vi "ReflectiveFunc.vi"(0 "Y":dbl[](array[numeric]), 1 "X":dbl[](array[numeric]), 2 "Coefficients":dbl[](array[numeric])) -> (3 "Y converted":dbl[](array[numeric]), 4 "X converted":dbl[](array[numeric]), 5 "Residue":dbl[](array[numeric]), 6 "f(X,a)":dbl[](array[numeric]))   [LabVIEW 2020, in "XYcenter.lvlib"]
uses:
  XYcenter.lvlib
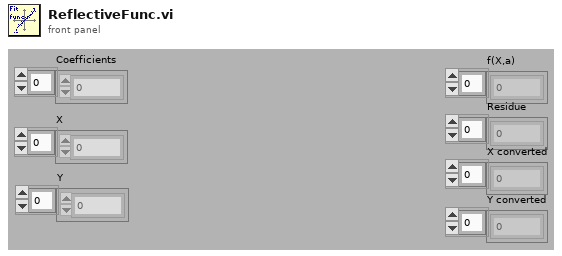
[diagram p1: front panel]
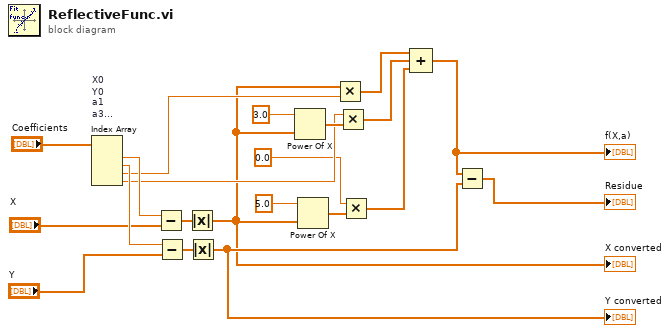
[diagram p0: block diagram]
diagram:
  n1 = Index Array "X0\nY0\na1\na3\na5"(array="Coefficients") -> (element #1=w17:dbl, element #2=w18:dbl, element #3=w7:dbl, element #4=w6:dbl)  [unwired: 4 in]
  n2 = Subtract(x=w17, y="X") -> (x-y=w20:dbl[])
  n3 = Subtract(x=w18, y="Y") -> (x-y=w19:dbl[])
  n4 = Absolute Value(x=w20) -> (abs(x)=w2:dbl[])
  "X converted" <- w2
  n5 = Absolute Value(x=w19) -> (abs(x)=w11:dbl[])
  "Y converted" <- w11
  n6 = Power Of X(1:w2, 2:3.0) -> (0:w15:dbl[])
  n7 = Power Of X(1:w2, 2:5.0) -> (0:w4:dbl[])
  n8 = Multiply(x=w2, y=w7) -> (x*y=w14:dbl[])
  n9 = Multiply(x=w6, y=w15) -> (x*y=w8:dbl[])
  n10 = Multiply(x=0.0, y=w4) -> (x*y=w3:dbl[])
  n11 = Compound Arithmetic op=ADD(w14, w8, w3) -> (w9:dbl[])
  "f(X,a)" <- w9
  n12 = Subtract(x=w9, y=w11) -> (x-y=→"Residue":dbl[])
